vi "set glyphArray.vi"(8 "error in (no error)":errorcluster, 10 "glyphArray":string[](array[string]), 11 "xceRootNode in":refnum<class "xceRootNode.lvclass">) -> (0 "error out":errorcluster, 3 "xceRootNode out":refnum<class "xceRootNode.lvclass">)   [LabVIEW 2013, in "xceRootNode.lvclass"]
uses:
  xceRootNode.lvclass
  xceRootNode.lvclass/xceRootNode.ctl
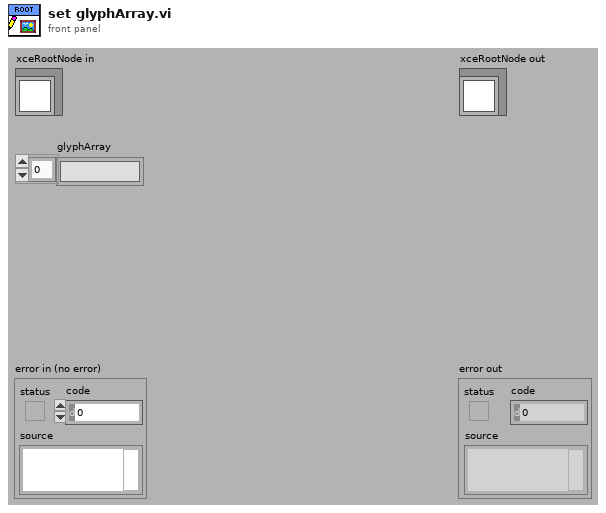
[diagram p1: front panel]
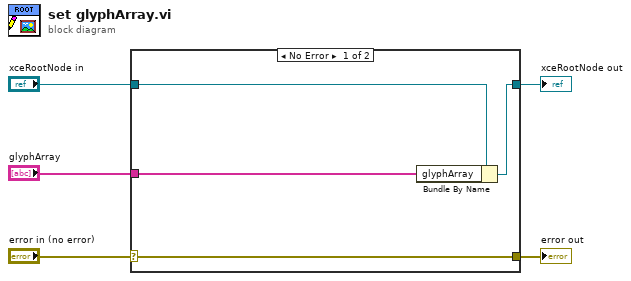
[diagram p0: block diagram]
diagram:
  n1 = case shown="No Error" "error in (no error)" {
    selector: "error in (no error)" -> [w9 w10]
    tunnel: [w9 w10] -> w4
    tunnel: [w7 w11] -> w2
    tunnel: "xceRootNode in" -> [w8 w11]
    tunnel: "glyphArray" -> [w6 _]
    frame No Error {
      n2 = Bundle By Name(cluster=w8, "glyphArray"=w6) -> (w7:refnum<class "xceRootNode.lvclass">)
    }
    frame Error {
    }
  }
  "error out" <- w4
  "xceRootNode out" <- w2
